vi "XYZ-TESTER-Main.vi"() -> ()   [LabVIEW 2020]
uses:
  _Core/Core-CtrlRefs.ctl
panel:
  out "T1":dbl(slide)=51.904761904761905 caption="温度1" scale=0.0..100.0
  out "T2":dbl(slide)=113.57142857142857 caption="温度2" scale=0.0..150.0
  out "Curv":cluster{dbl, dbl, dbl}(graph)
  in  "DAQSetting":bool
  in  "DAQRecord":bool
  out "LD.T2":string caption="后轴温度"
  out "LD.T3":string caption="绕组温度"
  out "LD.T1":string caption="前轴温度"
  out "LD.P":string caption="功率"
  out "LD.N":string caption="扭矩"
  out "LD.S":string caption="转速"
  out "Drv.T2":string caption="后轴温度"
  out "Drv.T3":string caption="绕组温度"
  out "Drv.T1":string caption="前轴温度"
  out "Drv.P":string caption="功率"
  out "Drv.N":string caption="扭矩"
  in  "AlarmClr":bool
  in  "PauseDAQ":bool
  in  "StartDAQ":bool
  in  "Exit":bool
  out "Alarm":i32(listbox) caption="日志报警"
  in  "TabCtrl":enum32{"手动控制", "自动控制", "数据记录"}(tab)
  in  "剩余时间(HH:MM:SS):":timestamp format="%< %H:%M:%S>T"
  in  "已运行时间(HH:MM:SS):":timestamp format="%< %H:%M:%S>T"
  in  "AdjL":bool
  in  "AdjV":bool
  in  "电加热":bool
  in  "淋水":bool
  in  "冷却泵":bool
  in  "油泵2":bool
  in  "油泵1":bool
  in  "加载运行":bool
  in  "驱动运行":bool
  in  "加载风机":bool
  in  "驱动风机":bool
  in  "调速速率":i32=50
  in  "驱动端转速":i32 max=6000 format="%#.0f"
  in  "调载速率":i32=10
  in  "加载端扭矩":i32
  in  "总运行时间(HH:MM:SS):":timestamp format="%< %H:%M:%S>T"
  in  "CtrlState":bool caption="控制:"
  in  "TestCtrl":bool caption="试验:"
  in  "StartMethod":enum32{"1Cycle", "allCycle"}(radio) caption="开始方式"
  in  "CycleMthod":enum32{"1Cycle", "allCycle"}(radio) caption="循环方式"
  in  "LoadPlot":i32(listbox) caption="荷载谱"
  in  "TData":i32(listbox) caption="测试数据"
  in  "TFile":i32(listbox) caption="测试文件"
  in  "EB":bool
  out "Drv.V":string caption="转速"
  in  "Ctrl-Refs":T1
  # "数据采集"
  # "驱动电机"
  # "XYZ TESTER \nVER: 1.0\ngaoke.yang@yahoo.com"
  # "加载电机"
  # "日志报警"
  # "驱动调速"
  # "荷载调速"
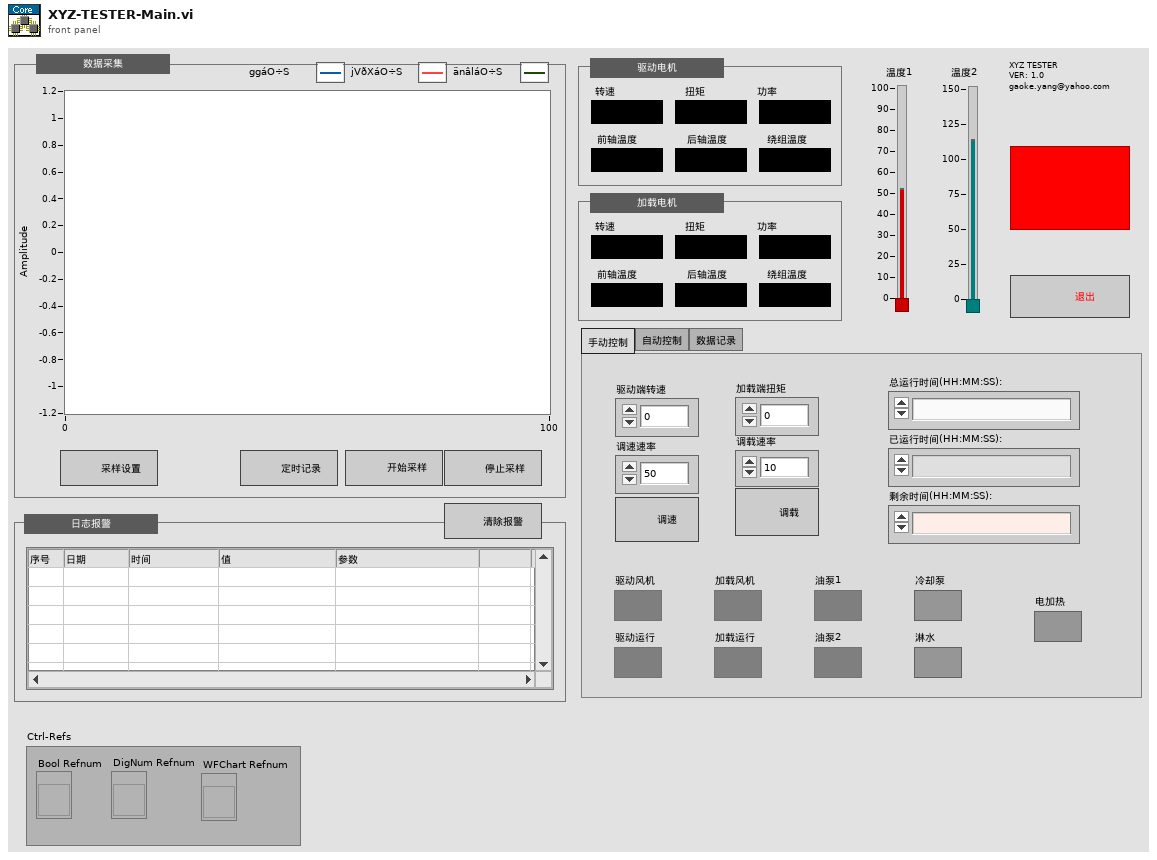
[diagram p1: front panel]
types:
  T1 = typedef "Core-CtrlRefs.ctl" = cluster{"Bool Refnum":refnum<vi>, "DigNum Refnum":refnum<vi>, "WFChart Refnum":refnum<vi>}
  T2 = cluster{"GUI::Initialize":refnum<user-event>, "GUI::User1":refnum<user-event>}
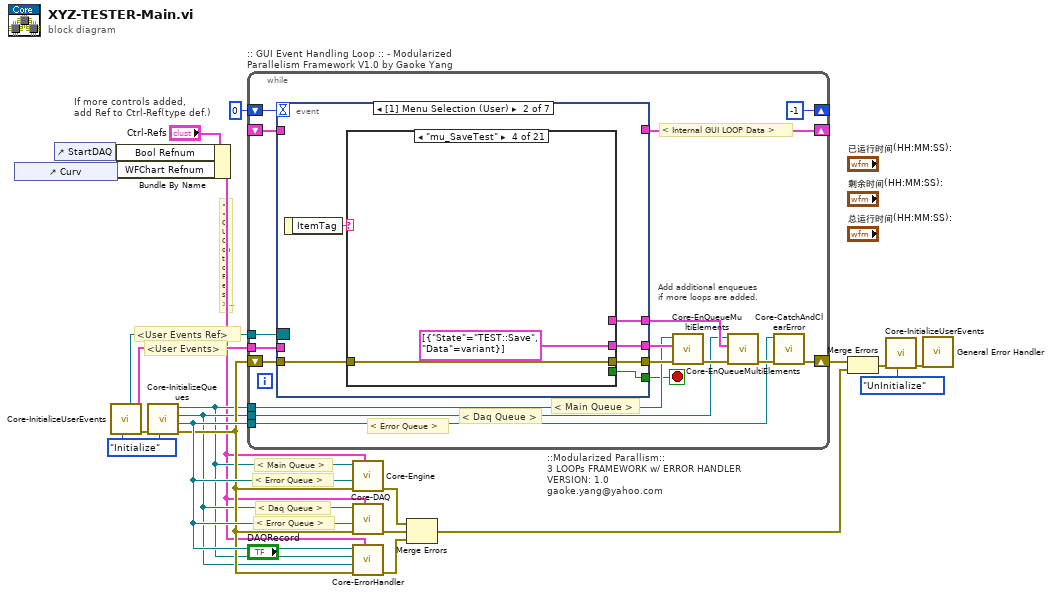
[diagram p0: block diagram]
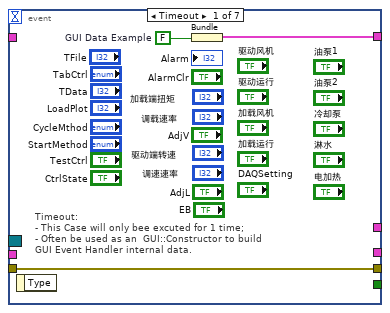
[diagram p2: hidden frame]
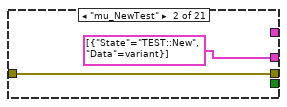
[diagram p4: hidden frame]
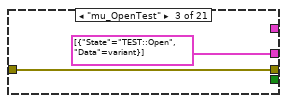
[diagram p5: hidden frame]
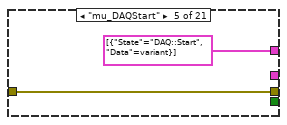
[diagram p6: hidden frame]
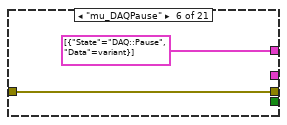
[diagram p7: hidden frame]
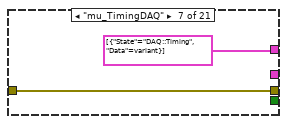
[diagram p8: hidden frame]
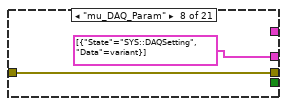
[diagram p9: hidden frame]
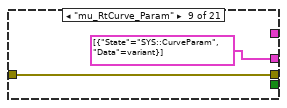
[diagram p10: hidden frame]
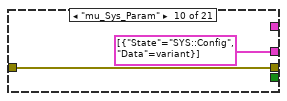
[diagram p11: hidden frame]
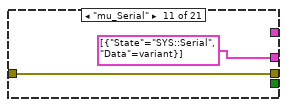
[diagram p12: hidden frame]
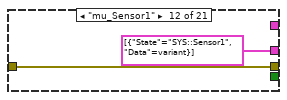
[diagram p13: hidden frame]
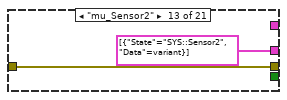
[diagram p14: hidden frame]
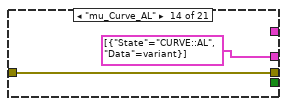
[diagram p15: hidden frame]
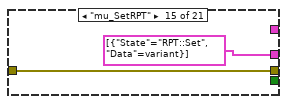
[diagram p16: hidden frame]
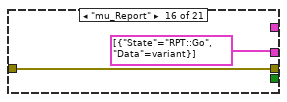
[diagram p17: hidden frame]
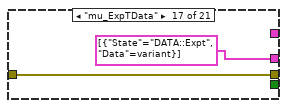
[diagram p18: hidden frame]
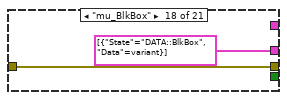
[diagram p19: hidden frame]
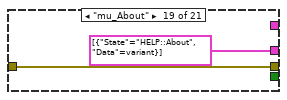
[diagram p20: hidden frame]
diagram:
  w18 = enum16{"Initialize", "UnInitialize"}."Initialize" ("Cmd(Initialize)")
  # "< Error Queue >"
  # "< Daq Queue >"
  # "< Error Queue >"
  # "< Main Queue >"
  # "If more controls added, \nadd Ref to Ctrl-Ref(type def.)"
  # "<< GUI Control Refs >>"
  # "<User Events>"
  # "<User Events Ref>"
  # "::Modularized Parallism::\n3 LOOPs FRAMEWORK w/ ERROR HANDLER\nVERSION: 1.0\ngaoke.yang@yahoo.com"
  n1 = control-ref of="Curv"() -> (w1:refnum<vi>)
  n2 = control-ref of="StartDAQ"() -> (w2:refnum<vi>)
  n3 = call "Core-InitializeUserEvents.vi"("Cmd(Initialize)"=w18) -> ("ErrO"=w19:errorcluster, "User Events"=w17:T2, "User Events\nRefnum"=w9:refnum<event-registration>)  [unwired: 8 in]
  n4 = Bundle By Name(cluster="Ctrl-Refs", "Bool Refnum"=w2, "WFChart Refnum"=w1) -> (w7:T1)
  n5 = call "Core-InitializeQueues.vi"("Cmd(Initialize)"=w18, "ErrI(No Error)"=w19) -> ("ErrO"=w12:errorcluster, "ErrQRef"=w13:refnum<queue>, "DaqQRef"=w11:refnum<queue>, "MainQRef"=w10:refnum<queue>)  [unwired: 6 in]
  n6 = while ":: GUI Event Handling Loop :: - Modularized Parallelism Framework V1.0 by Gaoke Yang" {
    tunnel: w10 -> [w34]
    shift-right: [w28] -> w20
    shift-left: w12 -> [w38]
    tunnel: w11 -> [w31]
    tunnel: w17 -> [w22]
    tunnel: w13 -> [w29]
    tunnel: w9 -> [w23]
    shift-right: [-1] -> _
    shift-left: 0 -> [w26]
    shift-right: [w25] -> _
    shift-left: _ -> [w24]
    stop <- w32 stop-if-true
    # "< Internal GUI LOOP Data >"
    # "Add additional enqueues \nif more loops are added."
    # "< Main Queue >"
    # "< Error Queue >"
    # "< Daq Queue >"
    n7 = event shown="[1] Menu Selection (User)" {
      selector: w23 -> [_ _ _ _ _ _ _]
      dyn-events: _ -> [_ _ _ _ _ _ _]
      timeout: w26 -> [_ _ _ _ _ _ _]
      tunnel: [_ w42 _ _ _ _ "Exit"] -> w32
      tunnel: w38 -> [w41 w45 w98 w100 w103 w104 w109]
      tunnel: [w41 w44 w98 w100 w103 w104 w108] -> w36
      tunnel: [_ w46 _ _ _ _ cluster{"State":string, "Data":variant}[] [{"State"="CMD::Exit", "Data"=variant}]] -> w37
      tunnel: [_ w43 _ _ cluster{"State":string, "Data":variant}[] [{"State"="DAQ::Start", "Data"=variant}] cluster{"State":string, "Data":variant}[] [{"State"="DAQ::Pause", "Data"=variant}] cluster{"State":string, "Data":variant}[] [{"State"="DAQ::Exit", "Data"=variant}]] -> w33
      tunnel: [w39 _ w97 w99 w101 _ w106] -> w25
      tunnel: w24 -> [_ _ w97 w99 w101 _ w106]
      tunnel: w22 -> [_ _ _ _ _ _ _]
      event Timeout {
        w40 = FALSE  # GUI Data Example
        # "Timeout:\n- This Case will only bee excuted for 1 time;\n- Often be used as an  GUI::Constructor to build\nGUI Event Handler internal data."
        n8 = event-data() -> ()  [unwired: 2 out]
        n9 = Bundle("GUI Data Example"=w40) -> (w39:cluster{"GUI Data Example":bool})  [unwired: 1 in]
      }
      event Menu Selection (User) {
        n10 = event-data() -> ("ItemTag"=w47:string)  [unwired: 1 out]
        n11 = case shown="\"mu_SaveTest\"" w47 {
          tunnel: [_ cluster{"State":string, "Data":variant}[] [{"State"="TEST::New", "Data"=variant}] cluster{"State":string, "Data":variant}[] [{"State"="TEST::Open", "Data"=variant}] cluster{"State":string, "Data":variant}[] [{"State"="TEST::Save", "Data"=variant}] _ _ _ cluster{"State":string, "Data":variant}[] [{"State"="SYS::DAQSetting", "Data"=variant}] cluster{"State":string, "Data":variant}[] [{"State"="SYS::CurveParam", "Data"=variant}] cluster{"State":string, "Data":variant}[] [{"State"="SYS::Config", "Data"=variant}] cluster{"State":string, "Data":variant}[] [{"State"="SYS::Serial", "Data"=variant}] cluster{"State":string, "Data":variant}[] [{"State"="SYS::Sensor1", "Data"=variant}] cluster{"State":string, "Data":variant}[] [{"State"="SYS::Sensor2", "Data"=variant}] cluster{"State":string, "Data":variant}[] [{"State"="CURVE::AL", "Data"=variant}] cluster{"State":string, "Data":variant}[] [{"State"="RPT::Set", "Data"=variant}] cluster{"State":string, "Data":variant}[] [{"State"="RPT::Go", "Data"=variant}] cluster{"State":string, "Data":variant}[] [{"State"="DATA::Expt", "Data"=variant}] cluster{"State":string, "Data":variant}[] [{"State"="DATA::BlkBox", "Data"=variant}] cluster{"State":string, "Data":variant}[] [{"State"="HELP::About", "Data"=variant}] cluster{"State":string, "Data":variant}[] [{"State"="HELP::Service", "Data"=variant}] cluster{"State":string, "Data":variant}[] [{"State"="CMD::Exit", "Data"=variant}]] -> w46
          tunnel: [w48 w49 w51 w54 w55 w58 w60 w62 w64 w66 w68 w70 w72 w74 w76 w78 w80 w82 w84 w86 w91] -> w44
          tunnel: w45 -> [w48 w49 w51 w54 w55 w58 w60 w62 w64 w66 w68 w70 w72 w74 w76 w78 w80 w82 w84 w86 w90]
          tunnel: [_ _ _ _ cluster{"State":string, "Data":variant}[] [{"State"="DAQ::Start", "Data"=variant}] cluster{"State":string, "Data":variant}[] [{"State"="DAQ::Pause", "Data"=variant}] cluster{"State":string, "Data":variant}[] [{"State"="DAQ::Timing", "Data"=variant}] _ _ _ _ _ _ _ _ _ _ _ _ _ cluster{"State":string, "Data":variant}[] [{"State"="DAQ::Exit", "Data"=variant}]] -> w43
          tunnel: [_ _ _ _ _ _ _ _ _ _ _ _ _ _ _ _ _ _ _ _ TRUE] -> w42
          frame Default {
          }
          frame "mu_NewTest" {
          }
          frame "mu_OpenTest" {
          }
          frame "mu_SaveTest" {
          }
          frame "mu_DAQStart" {
          }
          frame "mu_DAQPause" {
          }
          frame "mu_TimingDAQ" {
          }
          frame "mu_DAQ_Param" {
          }
          frame "mu_RtCurve_Param" {
          }
          frame "mu_Sys_Param" {
          }
          frame "mu_Serial" {
          }
          frame "mu_Sensor1" {
          }
          frame "mu_Sensor2" {
          }
          frame "mu_Curve_AL" {
          }
          frame "mu_SetRPT" {
          }
          frame "mu_Report" {
          }
          frame "mu_ExpTData" {
          }
          frame "mu_BlkBox" {
          }
          frame "mu_About" {
          }
          frame "mu_Service" {
          }
          frame "mu_Exit" {
            n12 = Bundle By Name(cluster=w90, "code"=9999) -> (w91:errorcluster)
          }
        }
      }
      event User Event {
        w96 = "" ("LD.S")
        # "User defined \"GUI::Initialize\" event handler:\nUse this case to initialize the GUI"
        n13 = event-data() -> ()  [unwired: 2 out]
        "Drv.N" <- w96
        "Drv.T3" <- w96
        "Drv.V" <- w96
        "Drv.P" <- w96
        "Drv.T1" <- w96
        "Drv.T2" <- w96
        "LD.S" <- w96
        "LD.N" <- w96
        "LD.P" <- w96
        "LD.T1" <- w96
        "LD.T3" <- w96
        "LD.T2" <- w96
        "Curv" <- cluster{dbl, dbl, dbl} {0.0, 0.0, 0.0} ("output cluster")
        "T2" <- 120.0 ("T2")
        "T1" <- 51.0 ("温度1")
      }
      event User Event {
        # "User defined \"GUI::User1\" event handler\nUse this case to handle user defined event."
        n14 = event-data() -> ()  [unwired: 2 out]
      }
      event "StartDAQ": Value Change {
        n15 = event-data() -> ()  [unwired: 2 out]
      }
      event "PauseDAQ": Value Change {
        n16 = event-data() -> ()  [unwired: 2 out]
      }
      event "Exit": Value Change; Panel Close {
        # "Exit Application:\n- Send Exit commands to Engine and Daq Loop;\n- Set error code to 9999 to close Error handling Loop.\nNotes:\n- User Defined Error Code Range are: 5000~9999(for Warnings) & -8999~-8000(For errors)"
        n17 = event-data() -> ()  [unwired: 2 out]
        n18 = Bundle By Name(cluster=w109, "code"=9999) -> (w108:errorcluster)
      }
    }
    n19 = call "Core-EnQueueMultiElements.vi"("ErrorIn"=w36, "CmdArray"=w37, "QRefIn"=w34) -> ("ErrorOut"=w35:errorcluster)  [unwired: 8 in]
    n20 = call "Core-EnQueueMultiElements.vi"("ErrorIn"=w35, "CmdArray"=w33, "QRefIn"=w31) -> ("ErrorOut"=w30:errorcluster)  [unwired: 8 in]
    n21 = call "Core-CatchAndClearError.vi"("Err-I"=w30, "ErrQ-I"=w29) -> ("Err-O"=w28:errorcluster)  [unwired: 9 in]
  }
  n22 = call "Core-Engine.vi"("Ctrl-Refs"=w7, "Err-I"=w12, "ErrQRef"=w13, "MainQ-I"=w10) -> ("Err-O"=w6:errorcluster)  [unwired: 7 in]
  n23 = call "Core-DAQ.vi"("Ctrl-Refs"=w7, "Err-I"=w12, "ErrQRef"=w13, "DaqQ-I"=w11) -> ("Err-O"=w5:errorcluster)  [unwired: 7 in]
  n24 = call "Core-ErrorHandler.vi"("Ctrl-Refs"=w7, "Err-I"=w12, "DaqQ-I"=w11, "MainQ-I"=w10, "ErrQ-I"=w13) -> ("Err-O"=w4:errorcluster)  [unwired: 6 in]
  n25 = Merge Errors(w6, w5, w4) -> (w3:errorcluster)
  n26 = Merge Errors(w20, w3) -> (w15:errorcluster)
  n27 = call "Core-InitializeUserEvents.vi"("Cmd(Initialize)"=enum16{"Initialize", "UnInitialize"}."UnInitialize", "ErrI(No Error)"=w15) -> ("ErrO"=w14:errorcluster)  [unwired: 7 in, 2 out]
  n28 = call <vilib>:"General Error Handler.vi"("error in (no error)"=w14) -> ()  [unwired: 10 in, 5 out]
